vi "ni5660 Sub Multi-Span FFT.vi"(0 "SMT zoom settings":T3 {"Frequency Shift" format="%.2f"; "zoom FFT settings"."zoom settings"."trim" format="%.2f"; "zoom FFT settings"."zoom settings"."center frequency" format="%.2f"}, 1 "restart averaging?":bool, 5 "Tuner Frequency Shift":dbl format="%.2f", 7 "DDC Frequency Shift":dbl format="%.2f", 9 "waveform":T4(array[cluster]) {"wfm" format="%.2f"; "xIncrement" format="%.2f"; "relativeInitialX" format="%.2f"}, 11 "error in (no error)":errorcluster, 12 "averaging parameters":T1={"averaging type"=enum."no averaging", "averaging settings"={"weighting type"=enum."linear", "weighting settings"={"size"=10.0, "linear weighting mode"=enum."moving average"}}}, 13 "fc adjust":dbl min=-0.5 max=0.5 format="%.2f") -> (4 "averaged FFT spectrum":cluster{"f0":dbl, "df":dbl, "spectrum":cdb[]} {"spectrum" format="%.2f"; "df" format="%.2f"; "f0" format="%.2f"}, 8 "data ready?":bool, 10 "spectral info in":T2, 14 "averages sofar":dbl, 15 "error out":errorcluster)   [LabVIEW 2011]
doc: "This example computes a corrected FFT spectrum for a span wider than 20 MHz. configures the RFSA to acquire a signal and compute a spectrum corresponding to a span wider than 20 MHz. This VI is a sub-VI of the RFSA Multi-Span Application VI."
uses:
  <vilib>/Analysis/sml.llb/aal_Complex Modulator(real input).vi
  <vilib>/Analysis/sml.llb/aal_Complex Modulator(complex input).vi
  <vilib>/Analysis/NI_AALPro.lvlib
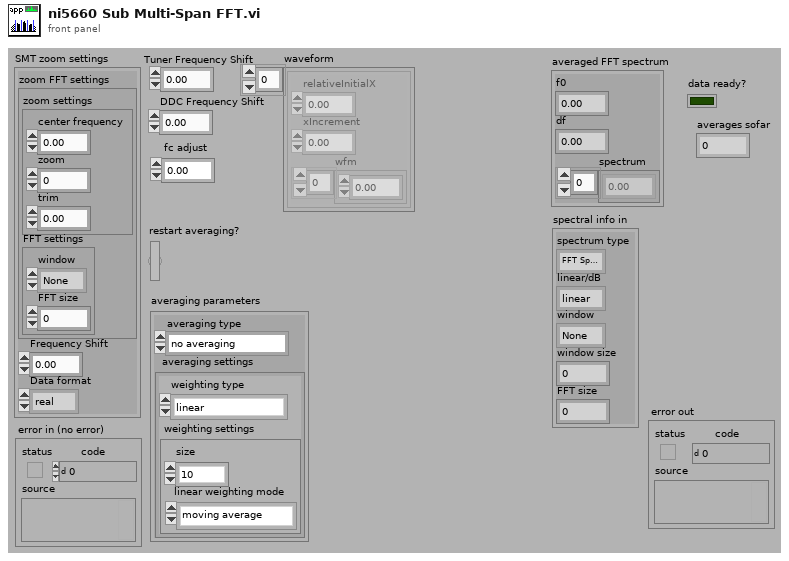
[diagram p1: front panel]
types:
  T1 = cluster{"averaging type":enum16{"no averaging", "vector averaging", "RMS averaging", "peak hold"}, "averaging settings":cluster{"weighting type":enum16{"linear", "exponential"}, "weighting settings":cluster{"size":dbl, "linear weighting mode":enum16{"one shot", "auto restart one shot", "moving average", "continuous"}}}}
  T2 = cluster{"spectrum type":enum16{"FFT Spectrum [complex]", "Amplitude [Magnitude]", "Power [Magnitude^2]", "Cross Spectrum [complex]", "Frequency Response [Complex]"}, "linear/dB":enum16{"linear", "dB"}, "window":enum16{"None ", "Hanning", "Hamming", "Blackman-Harris", "Exact Blackman", "Blackman", "Flat Top", "4 Term B-Harris ", "7 Term B-Harris", "Low Sidelobe"}, "window size":i32, "FFT size":i32}
  T3 = cluster{"zoom FFT settings":cluster{"zoom settings":cluster{"center frequency":dbl, "zoom":i32, "trim":dbl}, "FFT settings":cluster{"window":enum16{"None ", "Hanning", "Hamming", "Blackman-Harris", "Exact Blackman", "Blackman", "Flat Top", "4 Term B-Harris ", "7 Term B-Harris", "Low Sidelobe"}, "FFT size":i32}}, "Frequency Shift":dbl, "Data format":enum16{"real", "complex modulated (array)", "complex modulated (interleaved)"}}
  T4 = cluster{"relativeInitialX":dbl, "xIncrement":dbl, "wfm":dbl[]}[]
  T5 = enum16{"real", "complex modulated (array)", "complex modulated (interleaved)"}
  T6 = cluster{"relativeInitialX":dbl, "xIncrement":dbl, "wfm":dbl[]}
  T7 = typedef "NI_MAPro.lvlib/ma_sml_Spectral Info.ctl" = cluster{"spectrum type":enum16{"FFT Spectrum [complex]", "Amplitude [Magnitude]", "Power [Magnitude^2]", "Cross Spectrum [complex]", "Frequency Response [Complex]"}, "linear/dB":enum16{"linear", "dB"}, "window":u16, "window size":i32, "FFT size":i32}
  T8 = typedef "NI_MAPro.lvlib/ma_sml_Spectrum Cluster (complex).ctl" = cluster{"f0":dbl, "df":dbl, "spectrum":cdb[]}
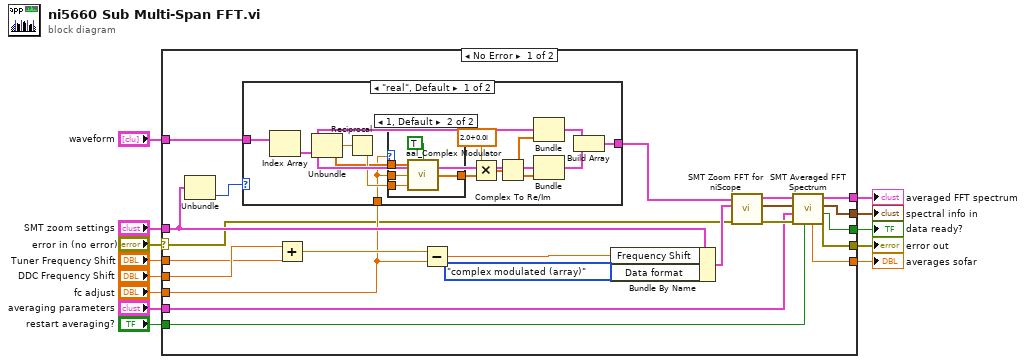
[diagram p0: block diagram]
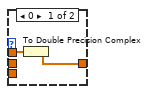
[diagram p2: hidden frame]
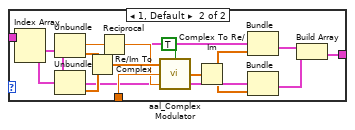
[diagram p4: hidden frame]
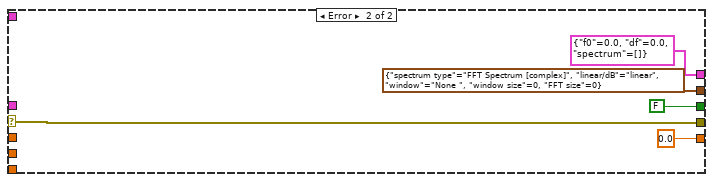
[diagram p5: hidden frame]
diagram:
  n1 = case shown="No Error" "error in (no error)" {
    selector: "error in (no error)" -> [w24 w81]
    tunnel: "SMT zoom settings" -> [w32 _]
    tunnel: "waveform" -> [w30 _]
    tunnel: "fc adjust" -> [w27 _]
    tunnel: "DDC Frequency Shift" -> [w26 _]
    tunnel: "Tuner Frequency Shift" -> [w25 _]
    tunnel: "restart averaging?" -> [w16 _]
    tunnel: [w17 0.0 ("averages sofar")] -> w7
    tunnel: [w21 w81] -> w6
    tunnel: [w20 FALSE ("data ready?")] -> w5
    tunnel: [w19 T2 {"spectrum type"=enum."FFT Spectrum [complex]", "linear/dB"=enum."linear", "window"=enum."None ", "window size"=0, "FFT size"=0} ("spectral info out")] -> w4
    tunnel: [w18 cluster{"f0":dbl, "df":dbl, "spectrum":cdb[]} {"f0"=0.0, "df"=0.0, "spectrum"=[]} ("averaged FFT spectrum")] -> w3
    tunnel: "averaging parameters" -> [w14 _]
    frame No Error {
      n2 = Unbundle(w32) -> ("Data format"=w31:T5)  [unwired: 2 out]
      n3 = case shown="\"real\", Default" w31 {
        tunnel: w30 -> [w49 w59]
        tunnel: w27 -> [w39 w57]
        tunnel: [w42 w58] -> w29
        frame "real", Default {
          n4 = Index Array(array=w49) -> (element=w48:T6)  [unwired: 1 in]
          n5 = Unbundle(w48) -> ("xIncrement"=w47:dbl, "wfm"=w45:dbl[])  [unwired: 1 out]
          n6 = Reciprocal(x=w47) -> (1/x=w46:dbl)
          n7 = case shown="1, Default" w39 {
            tunnel: w46 -> [_ w56]
            tunnel: w45 -> [w51 w55]
            tunnel: w39 -> [_ w53]
            tunnel: [w50 w52] -> w38
            frame 0 {
              n8 = To Double Precision Complex(1:w51) -> (0:w50:cdb[])
            }
            frame 1, Default {
              n9 = call-poly <vilib>:"aal_Complex Modulator.vi"("reset ?"=TRUE, "fs"=w56, "frequency"=w53, "x"=w55) -> ("y"=w52:cdb[])
            }
          }
          n10 = Multiply(x=cdb 2.0+0.0i ("Numeric 2"), y=w38) -> (x*y=w37:cdb[])
          n11 = Complex To Re/Im(x + iy=w37) -> (x=w41:dbl[], y=w40:dbl[])
          n12 = Bundle(cluster=w48, "wfm"=w41) -> (w44:T6)  [unwired: 2 in]
          n13 = Bundle(cluster=w48, "wfm"=w40) -> (w43:T6)  [unwired: 2 in]
          n14 = Build Array(w44, w43) -> (w42:T4)
        }
        frame "complex modulated (array)" {
          n15 = case shown="0" w57 {
            tunnel: w59 -> [w60 w76]
            tunnel: w57 -> [_ w71]
            tunnel: [w60 w62] -> w58
            frame 0 {
            }
            frame 1, Default {
              n16 = Index Array(array=w76) -> (element #1=w66:T6, element #2=w75:T6)  [unwired: 2 in]
              n17 = Unbundle(w66) -> ("xIncrement"=w70:dbl, "wfm"=w74:dbl[])  [unwired: 1 out]
              n18 = Unbundle(w75) -> ("wfm"=w73:dbl[])  [unwired: 2 out]
              n19 = Re/Im To Complex(1:w73, 2:w74) -> (0:w72:cdb[])
              n20 = Reciprocal(x=w70) -> (1/x=w69:dbl)
              n21 = call-poly <vilib>:"aal_Complex Modulator.vi"("reset ?"=TRUE, "fs"=w69, "frequency"=w71, "x"=w72) -> ("y"=w67:cdb[])
              n22 = Complex To Re/Im(x + iy=w67) -> (x=w65:dbl[], y=w61:dbl[])
              n23 = Bundle(cluster=w66, "wfm"=w65) -> (w64:T6)  [unwired: 2 in]
              n24 = Bundle(cluster=w66, "wfm"=w61) -> (w63:T6)  [unwired: 2 in]
              n25 = Build Array(w64, w63) -> (w62:T4)
            }
          }
        }
      }
      n26 = Add(x=w26, y=w25) -> (x+y=w35:dbl)
      n27 = Subtract(x=w35, y=w27) -> (x-y=w28:dbl)
      n28 = Bundle By Name(cluster=w32, "Frequency Shift"=w28, "Data format"=T5."complex modulated (array)") -> (w34:T3)
      n29 = call <vilib>:"SMT Zoom FFT for niScope.vi"("error in (no error)"=w24, "SMT zoom settings"=w34, "waveforms"=w29) -> ("error out"=w15:errorcluster, "spectral info"=w22:T7, "FFT spectrum (Vrms)"=w23:T8)  [unwired: 6 in]
      n30 = call <vilib>:"SMT Averaged FFT Spectrum.vi"("restart averaging?"=w16, "error in (no error)"=w15, "averaging parameters"=w14, "spectral info in"=w22, "FFT spectrum"=w23) -> ("error out"=w21:errorcluster, "data ready?"=w20:bool, "spectral info out"=w19:T2, "averaged FFT spectrum"=w18:cluster{"f0":dbl, "df":dbl, "spectrum":cdb[]}, "averages so far"=w17:dbl)  [unwired: 2 in]
    }
    frame Error {
    }
  }
  "error out" <- w6
  "spectral info in" <- w4
  "averaged FFT spectrum" <- w3
  "data ready?" <- w5
  "averages sofar" <- w7
